vi "Shooter State Machine.vi"() -> ()   [LabVIEW 2011]
uses:
  Controls/Shooter Shifter.ctl
panel:
  in  "Shooter Speed":dbl
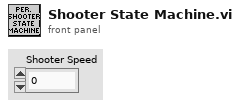
[diagram p1: front panel]
types:
  T1 = typedef "Shooter Shifter.ctl" = enum16{"Wait for button", "Align robot", "Accelerate shooter", "Feed ball"}
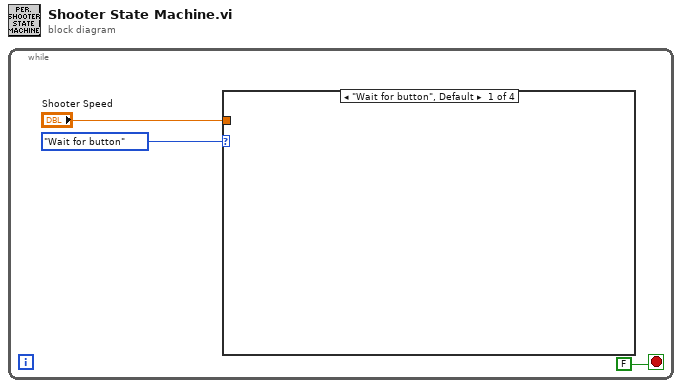
[diagram p0: block diagram]
diagram:
  n1 = while {
    stop <- FALSE stop-if-true
    n2 = case shown="\"Wait for button\", Default" Shooter_Shifter."Wait for button" {
      tunnel: "Shooter Speed" -> [_ _ _ _]
      frame "Wait for button", Default {
      }
      frame "Align robot" {
      }
      frame "Accelerate shooter" {
      }
      frame "Feed ball" {
      }
    }
  }
